vi "calc_running_avg.vi"(9 "Size of batch":u32, 10 "Averages in":dbl[](array[numeric]), 11 "Measure data":dbl[](array[numeric])) -> (3 "Averages out":dbl[](array[numeric]))   [LabVIEW 2022 SP3]
uses:
  <vilib>/Analysis/baseanly.llb/Mean (DBL).vi
  <vilib>/Analysis/NI_AALBase.lvlib
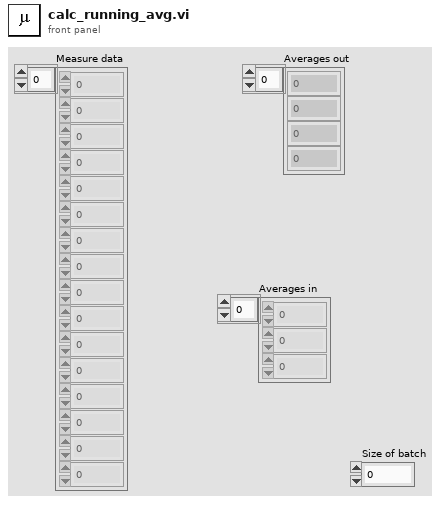
[diagram p1: front panel]
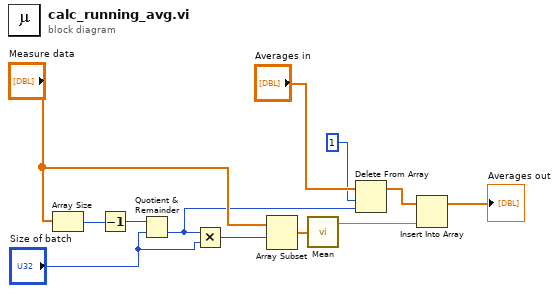
[diagram p0: block diagram]
diagram:
  n1 = Array Size(array="Measure data") -> (size(s)=w11:i32)
  n2 = Decrement(x=w11) -> (x-1=w1:i32)
  n3 = Quotient & Remainder(x=w1, y="Size of batch") -> (floor(x/y)=w7:u32)  [unwired: 1 out]
  n4 = Multiply(x=w7, y="Size of batch") -> (x*y=w2:u32)
  n5 = Array Subset(array="Measure data", index=w2) -> (w9:dbl[])  [unwired: 1 in]
  n6 = call-poly <vilib>:"Mean.vi"("X"=w9) -> ("mean"=w5:dbl)  [unwired: 1 out]
  n7 = Delete From Array(array="Averages in", length=1, index=w7) -> (array with subset deleted=w6:dbl[])  [unwired: 1 out]
  n8 = Insert Into Array(array=w6, new element=w5) -> (→"Averages out":dbl[])  [unwired: 1 in]
